vi "Material-Application-DeploymentConstants.vi"() -> ()   [LabVIEW 2013]
panel:
  in  "Deploy-App-Mutex":string="WirebirdLabsDeploy"
  in  "Deploy-App-FullName":string="Deploy v2013.1.0.1809"
  in  "Deploy-App-VersionShort":string="2013.1.0"
  in  "Deploy-App-Version":string="2013.1.0.1809"
  in  "Deploy-App-TaglinePublisher":string="Wirebird Labs: Expert Toolkits for LabVIEW™" caption="Wirebird Labs: Tagline"
  in  "Deploy-App-LegalCopyrightLong":string="Wirebird Labs: Deploy™ © 2012-2013 Wirebird Labs LLC. All rights reserved." caption="Wirebird Labs: Deploy Copyright (long)"
  in  "Deploy-App-LegalCopyright":string="Copyright © 2012-2013 Wirebird Labs LLC" caption="Wirebird Labs Copyright"
  in  "Deploy-App-DisplayName":string="Deploy"
  in  "Deploy-App-Publisher":string="Wirebird Labs LLC"
  # "Application"
  # "Copyrights"
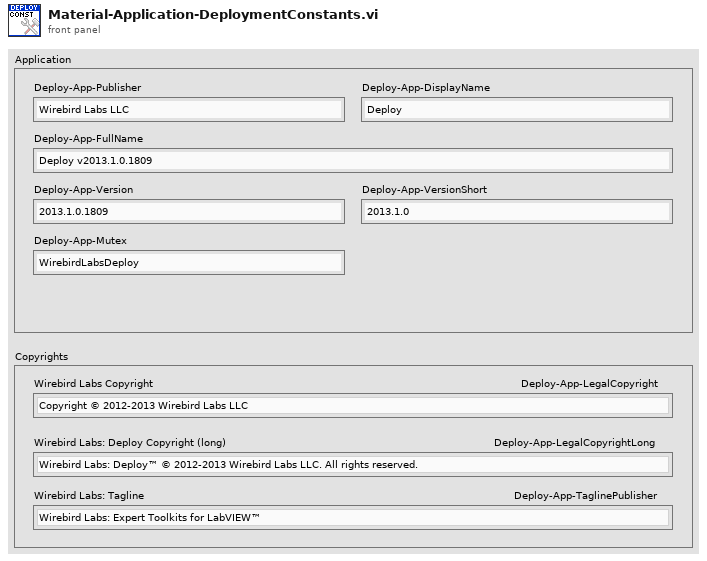
[diagram p1: front panel]
diagram:
